vi "Create Coverage Report - With Parent - Package Name Is Parent Qualified Name.vi"() -> ()   [LabVIEW 2017, in "Cobertura.Tests.lvlib"]
uses:
  Cobertura.Tests.lvlib
  Fake Code Coverage/Fake Code Coverage.lvclass
  C:/Users/pasca/Projects/Home/lvunit/CodeCoverage/CodeCoverage.lvclass
  Cobertura/Coverage/Coverage.lvclass/Coverage.ctl
  Cobertura/Package/Package.lvclass/Package.ctl
  Cobertura/Coverage/Read Packages.vi
  Cobertura/Package/Read Name.vi
  Fake Project Inspector/Fake Project Inspector.lvclass
  C:/Users/pasca/Projects/Home/lvunit/Cobertura/Project Inspector Base/Project Inspector Base.lvclass
  Fake Code Inspector/Fake Code Inspector.lvclass
  C:/Users/pasca/Projects/Home/lvunit/Cobertura/Code Inspector Base/Code Inspector Base.lvclass
  Cobertura/Package/Package.lvclass
  Cobertura/Cobertura.lvlib
  Cobertura/Coverage/Coverage.lvclass
  <vilib>/PNR/Transparent Assertions/Transparent Assertions/Transparent Assertions.lvlib
panel:
  out "error out":errorcluster
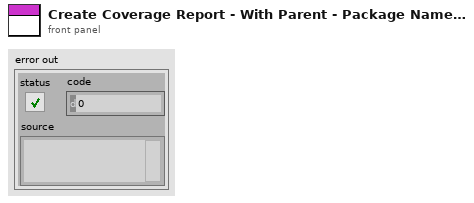
[diagram p1: front panel]
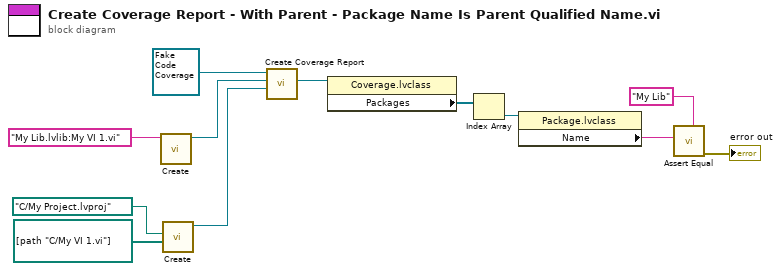
[diagram p0: block diagram]
diagram:
  n1 = call "Create.vi"("VI Name"="My Lib.lvlib:My VI 1.vi") -> ("Fake Code Inspector"=w2:refnum<class "Fake Code Inspector.lvclass">)  [unwired: 9 in, 1 out]
  n2 = call "Create.vi"("Item Paths"=path[] [path "C:/My VI 1.vi"], "Path"=path "C:/My Project.lvproj") -> ("Fake Project Inspector"=w8:refnum<class "Fake Project Inspector.lvclass">)  [unwired: 8 in, 1 out]
  n3 = call "Create Coverage Report.vi"("Project Inspector"=w8, "Code Inspector"=w2, "CodeCoverage in"=refnum<class "Fake Code Coverage.lvclass"> refnum ("Cobertura.Tests.lvlib:Fake Code Coverage.lvclass")) -> ("Coverage"=w12:refnum<class "Coverage.lvclass">)  [unwired: 7 in, 1 out]
  n4 = property class="Coverage.lvclass"(reference=w12) -> ("Packages"=w10:refnum<class "Package.lvclass">[])  [unwired: 1 in, 2 out]
  n5 = Index Array(array=w10) -> (element=w6:refnum<class "Package.lvclass">)  [unwired: 1 in]
  n6 = property class="Package.lvclass"(reference=w6) -> ("Name"=w5:string)  [unwired: 1 in, 2 out]
  n7 = call <vilib>:"Assert Equal.vi"("Expected"="My Lib", "Actual"=w5) -> ("error out"=→"error out":errorcluster)  [unwired: 9 in]
